vi "Get and sort visible controls.vi"(8 "error in (no error)":errorcluster, 11 "VI reference":refnum<vi>) -> (0 "error out":errorcluster, 1 "Ordered control labels":string[](array[string]), 2 "Visible control references":refnum<vi>[](array[refnum]), 3 "VI reference out":refnum<vi>)   [LabVIEW 2017, in "verticalDistribution.lvlib"]
uses:
  <vilib>/Utility/vertDist/verticalDistribution.lvlib
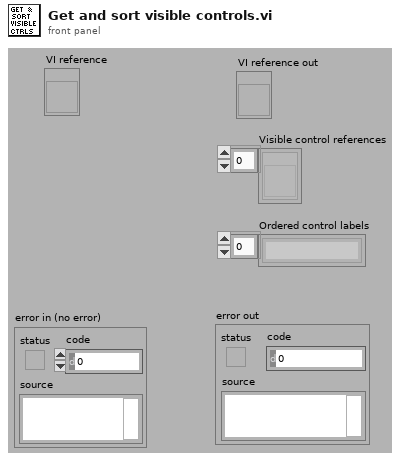
[diagram p1: front panel]
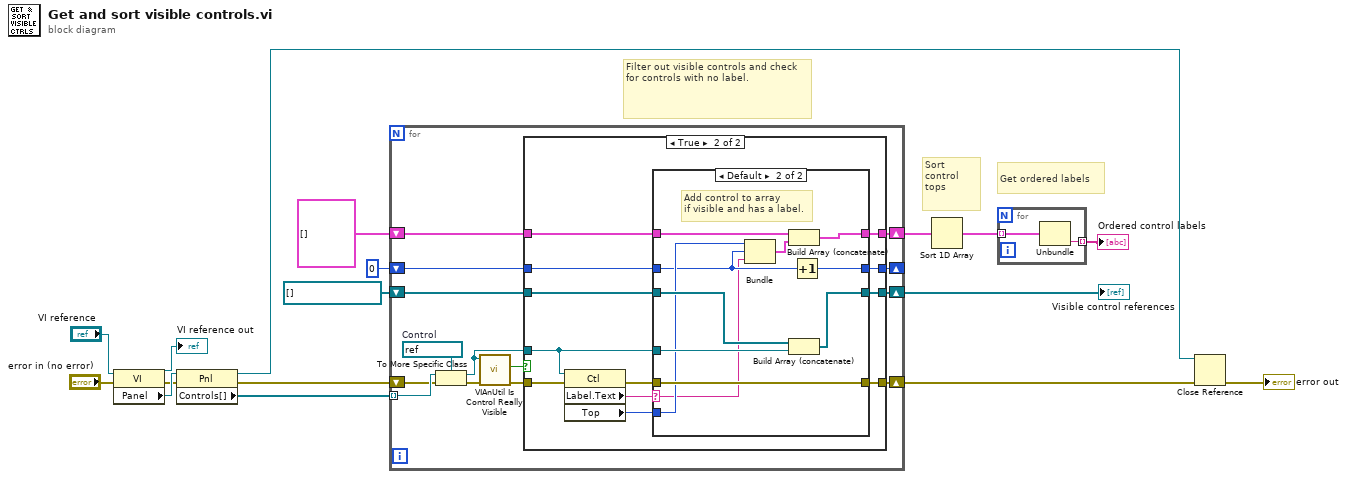
[diagram p0: block diagram]
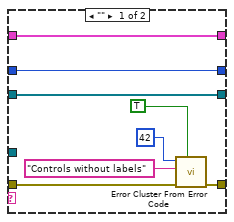
[diagram p3: hidden frame]
diagram:
  # "Filter out visible controls and check for controls with no label."
  # "Get ordered labels"
  # "Sort \ncontrol \ntops"
  n1 = property class="VI"(reference="VI reference", error in="error in (no error)") -> (reference out=→"VI reference out":refnum<vi>, error out=w16:errorcluster, "Panel"=w17:refnum<vi>)
  n2 = property class="Pnl"(reference=w17, error in=w16) -> (reference out=w15:refnum<vi>, error out=w9:errorcluster, "Controls[]"=w11:refnum<vi>[])
  n3 = for {
    tunnel: w11 -> [w30] mode=indexing
    shift-right: [w22] -> w3
    shift-left: w9 -> [w29]
    shift-right: [w28] -> w1
    shift-left: refnum<vi>[] [] -> [w27]
    shift-right: [w21] -> w8
    shift-left: cluster{"Top":i32, i32, string}[] [] -> [w20]
    shift-right: [w18] -> _
    shift-left: 0 -> [w19]
    w31 = refnum<vi> refnum  # Control
    n4 = To More Specific Class(target class=w31, reference=w30, error in=w29) -> (specific class reference=w24:refnum<vi>, error out=w26:errorcluster)
    n5 = call <vilib>:"VIAnUtil Is Control Really Visible.vi"("error in (no error)"=w26, "GObj Refnum"=w24) -> ("error out"=w23:errorcluster, "Control really visible?"=w25:bool)  [unwired: 8 out]
    n6 = case shown="True" w25 {
      tunnel: w24 -> [_ w45]
      tunnel: [w35 w47] -> w28
      tunnel: w27 -> [w35 w46]
      tunnel: w23 -> [w34 w43]
      tunnel: [w34 w41] -> w22
      tunnel: [w33 w39] -> w21
      tunnel: w20 -> [w33 w38]
      tunnel: w19 -> [w32 w37]
      tunnel: [w32 w36] -> w18
      frame False {
      }
      frame True {
        n7 = property class="Ctl"(reference=w45, error in=w43) -> (error out=w42:errorcluster, "Label.Text"=w44:string, "Top"=w40:i32)  [unwired: 1 out]
        n8 = case shown="Default" w44 {
          selector: w44 -> [_ w56]
          tunnel: [w50 w66] -> w47
          tunnel: w46 -> [w50 w65]
          tunnel: w45 -> [_ w64]
          tunnel: w42 -> [w52 w63]
          tunnel: [w51 w63] -> w41
          tunnel: w40 -> [_ w62]
          tunnel: [w49 w61] -> w39
          tunnel: w38 -> [w49 w59]
          tunnel: w37 -> [w48 w58]
          tunnel: [w48 w57] -> w36
          frame "" {
            n9 = call <vilib>:"Error Cluster From Error Code.vi"("show call chain? (False)"=TRUE, "error in (no error)"=w52, "error message (\"\")"="Controls without labels", "error code (0)"=42) -> ("error out"=w51:errorcluster)  [unwired: 5 out]
          }
          frame Default {
            # "Add control to array\nif visible and has a label."
            n10 = Bundle("Top"=w62, w58, w56) -> (w60:cluster{"Top":i32, i32, string})  [unwired: 1 out]
            n11 = Build Array (concatenate)(w59, w60) -> (w61:cluster{"Top":i32, i32, string}[])
            n12 = Build Array (concatenate)(w65, w64) -> (w66:refnum<vi>[])
            n13 = Increment(x=w58) -> (x+1=w57:i32)
          }
        }
      }
    }
  }
  "Visible control references" <- w1
  n14 = Sort 1D Array(array=w8) -> (sorted array=w6:cluster{"Top":i32, i32, string}[])
  n15 = for {
    tunnel: w6 -> [w68] mode=indexing
    tunnel: [w67] -> w4 mode=indexing
    n16 = Unbundle(w68) -> (w67:string)  [unwired: 2 out]
  }
  "Ordered control labels" <- w4
  n17 = Close Reference(reference=w15, error in (no error)=w3) -> (error out=→"error out":errorcluster)
